vi "SPD.Set Meas Grid.vi"(8 "Error In":errorcluster, 9 "HV_GridParams":T1, 10 "SPD.DCR Meas Setup":T12={"Strobe_code"={"Start"=0.0, "Stop"=0.0, "Step"=0.0}, "Temperature"={"Start"=-45.0, "Stop"=-45.0, "Step"=2.5}} caption="Настройка Измерений", 11 "SPD.Stand Ctrl in":T2 {"spdDeviceSession"."hidSPD.Controller"."HV_bias" format="%#_6p, V"; "spdDeviceSession"."hidSPD.Controller"."TSet" format="%#_6p, DegC"}) -> (0 "Error Out":errorcluster, 3 "SPD.Stand Ctrl out":T2 {"spdDeviceSession"."hidSPD.Controller"."HV_bias" format="%#_6p, V"; "spdDeviceSession"."hidSPD.Controller"."TSet" format="%#_6p, DegC"})   [LabVIEW 2018]
uses:
  SubTests/Measurements/SPD.Grid Meas Setup.ctl
  SubTests/Measurements/SPD.Test Range.ctl
  typedefs/SPD.Stand Ctrl.ctl
  Instruments/SPD HID Interface/hidSPDLibForLabView/LibVIs/hidSPD Controls/hidSPD Device Session.ctl
  Instruments/SPD HID Interface/hidSPDLibForLabView/LibVIs/hidSPD Controls/hidSPD Controller.ctl
  Instruments/KC705 DevBoard/typedefs/DevB.Session.ctl
  Instruments/KeySight 53230A/typedefs/FreqC.Session.ctl
  Instruments/KeySight 8164B/KeySight 8164B LAN InstrLib/typedefs/KeySight 8164B control.ctl
  Instruments/LeCroy SDA830/typedefs/LeCroy.Session.ctl
  typedefs/SPD.Events.ctl
  <vilib>/Utility/config.llb/Config Data RefNum.ctl
  typedefs/SPD.Meas Result.ctl
  SubTests/03_MeasGrid/SPD.HV_Grid Test Params.ctl
  <vilib>/Analysis/1siggen.llb/Ramp Pattern by Delta.vi
  <vilib>/Analysis/NI_AALBase.lvlib
  Instruments/SPD HID Interface/hidSPDLibForLabView/hidSPDLibForLabView.lvlib
  Instruments/KeySight 8164B/KeySight 8164B LAN InstrLib.lvlib
  <vilib>/Utility/config.llb/NI_LVConfig.lvlib
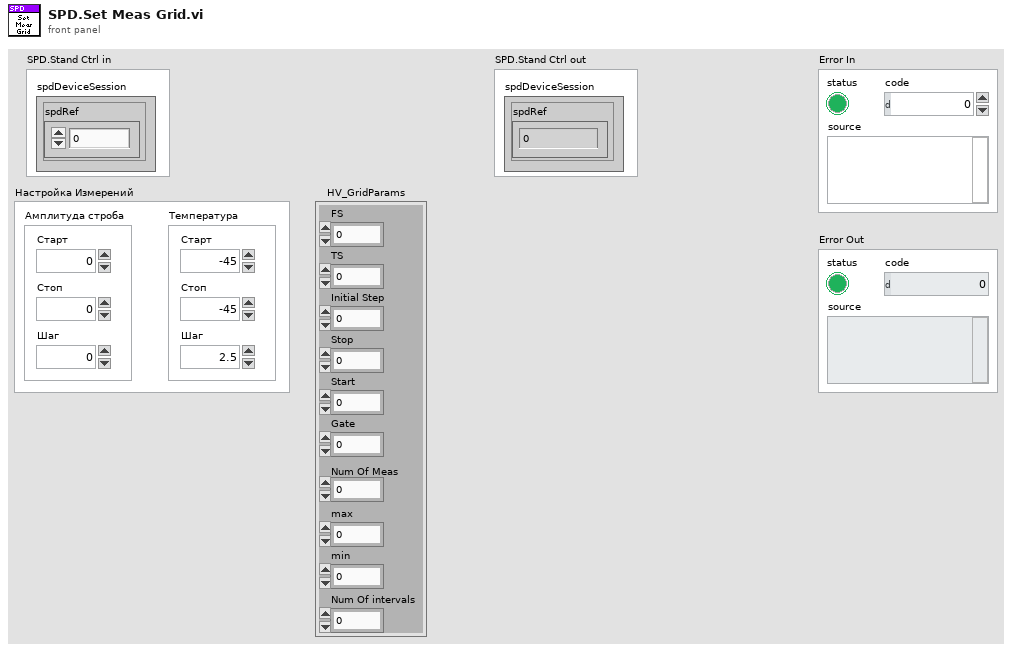
[diagram p1: front panel]
types:
  T1 = typedef "SPD.HV_Grid Test Params.ctl" = cluster{"FS":i32, "TS":i32, "Initial Step":dbl, "Stop":dbl, "Start":dbl, "Gate":dbl, "Num Of Meas":i32, "max":dbl, "min":dbl, "Num Of intervals":i32}
  T2 = typedef "SPD.Stand Ctrl.ctl" = cluster{"spdDeviceSession":T3, "DevBSession":T5, "FreqCSession":T6, "8164BSession":T7, "LeCroySession":T8, "Events":T9, "configFile":T10, "SPD.Result":T11}
  T3 = typedef "hidSPDLibForLabView.lvlib/hidSPD Device Session.ctl" = cluster{"spdRef":u64, "connected":bool, "spdName":string, "hidSPD.Controller":T4}
  T4 = typedef "hidSPDLibForLabView.lvlib/hidSPD Controller.ctl" = cluster{"TSet":sgl, "HV_bias":sgl, "DDS_stb_code":u16}
  T5 = typedef "DevB.Session.ctl" = cluster{"DevBRef":refnum<visa-resource-name>, "connected":bool}
  T6 = typedef "FreqC.Session.ctl" = cluster{"FreqCRef":refnum<visa-resource-name>, "timeout":dbl, "Gate":dbl, "connected":bool}
  T7 = typedef "KeySight 8164B LAN InstrLib.lvlib/KeySight 8164B control.ctl" = cluster{"Connection ID":refnum<k5>, "Connected":bool, "Info":string, "Slots Info":string[]}
  T8 = typedef "LeCroy.Session.ctl" = cluster{"LeCroySession":refnum<visa-resource-name>, "connected":bool}
  T9 = typedef "SPD.Events.ctl" = cluster{"DCRTest":refnum<user-event>, "Stop":refnum<user-event>}
  T10 = typedef "NI_LVConfig.lvlib/Config Data RefNum.ctl" = refnum<k1>
  T11 = typedef "SPD.Meas Result.ctl" = cluster{"HV_Bias":dbl[][][], "Stb_code":dbl[], "Temprature":dbl[], "Data":dbl[][][][]}
  T12 = typedef "SPD.Grid Meas Setup.ctl" = cluster{"Strobe_code":T13, "Temperature":T13}
  T13 = typedef "SPD.Test Range.ctl" = cluster{"Start":dbl, "Stop":dbl, "Step":dbl}
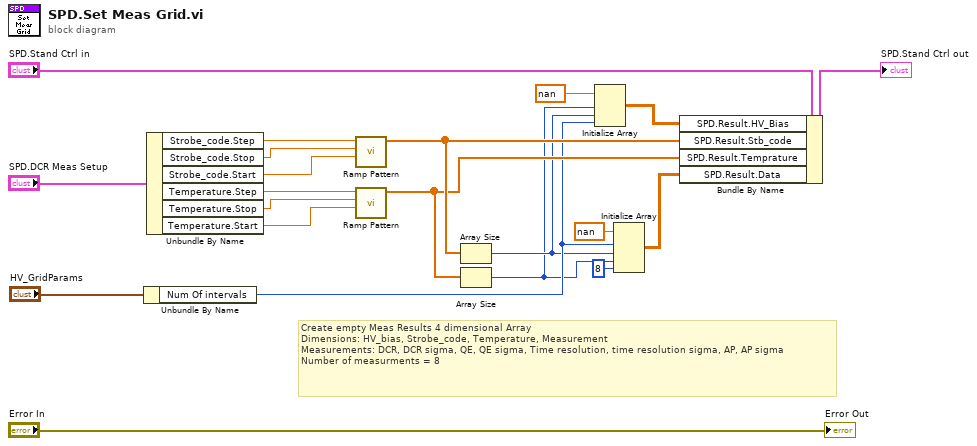
[diagram p0: block diagram]
diagram:
  # "Create empty Meas Results 4 dimensional Array\nDimensions: HV_bias, Strobe_code, Temperature, Measurement\nMeasurements: DCR, DCR sigma, QE, QE sigma, Time resolution, time resolution sigma, AP, AP sigma\nNumber of measurments = 8"
  n1 = Unbundle By Name("HV_GridParams") -> ("Num Of intervals"=w5:i32)
  n2 = Unbundle By Name("SPD.DCR Meas Setup") -> ("Strobe_code.Step"=w21:dbl, "Strobe_code.Stop"=w20:dbl, "Strobe_code.Start"=w19:dbl, "Temperature.Step"=w18:dbl, "Temperature.Stop"=w17:dbl, "Temperature.Start"=w16:dbl)
  n3 = call-poly <vilib>:"Ramp Pattern.vi"("start"=w19, "end"=w20, "delta"=w21) -> ("Ramp Pattern"=w10:dbl[])  [unwired: 6 in, 2 out]
  n4 = call-poly <vilib>:"Ramp Pattern.vi"("start"=w16, "end"=w17, "delta"=w18) -> ("Ramp Pattern"=w9:dbl[])  [unwired: 6 in, 2 out]
  n5 = Array Size(array=w10) -> (size(s)=w4:i32)
  n6 = Array Size(array=w9) -> (size(s)=w3:i32)
  n7 = Initialize Array(nan ("element"), w3, w4, w5) -> (w1:dbl[][][])
  n8 = Initialize Array(nan ("element"), w5, w4, w3, 8 ("dimension size")) -> (w6:dbl[][][][])
  n9 = Bundle By Name(cluster="SPD.Stand Ctrl in", "SPD.Result.HV_Bias"=w1, "SPD.Result.Stb_code"=w10, "SPD.Result.Temprature"=w9, "SPD.Result.Data"=w6) -> (→"SPD.Stand Ctrl out":T2)
  "Error Out" <- "Error In"
